vi "VISJS Viewer.vi"(4 "Extra Scripts":string, 5 "FileDependency out":map{path, T1}(c390), 6 "Options":string, 7 "OpenWebBrowser(False)":bool, 8 "error in":errorcluster, 9 "Embedd VISJS Librarya in HTMl File(False)":bool, 10 "HTMLFilePath":path, 11 "LibraryDependency":map{path, T3}(c390)) -> (0 "error out":errorcluster, 3 "HTMLFileContent":string)   [LabVIEW 2020, in "VISJS Viewer.lvlib"] (continued)
this.defaultOptions),this.body.emitter.on(\"_dataChanged\",(function(){e.updateSelection()}))}return kd(g,[{key:\"setOptions\",value:function(g){if(void 0!==g){Xf([\"multiselect\",\"hoverConnectedEdges\",\"selectable\",\"selectConnectedEdges\"],this.options,g)}}},{key:\"selectOnPoint\",value:function(g){var t=!1;if(!0===this.options.selectable){var A=this.getNodeAt(g)||this.getEdgeAt(g);this.unselectAll(),void 0!==A&&(t=this.selectObject(A)),this.body.emitter.emit(\"_requestRedraw\")}return t}},{key:\"selectAdditionalOnPoint\",value:function(g){var t=!1;if(!0===this.options.selectable){var A=this.getNodeAt(g)||this.getEdgeAt(g);void 0!==A&&(t=!0,!0===A.isSelected()?this.deselectObject(A):this.selectObject(A),this.body.emitter.emit(\"_requestRedraw\"))}return t}},{key:\"_initBaseEvent\",value:function(g,t){var A={};return A.pointer={DOM:{x:t.x,y:t.y},canvas:this.canvas.DOMtoCanvas(t)},A.event=g,A}},{key:\"generateClickEvent\",value:function(g,t,A,e){var C=arguments.length>4&&void 0!==arguments[4]&&arguments[4],I=this._initBaseEvent(t,A);if(!0===C)I.nodes=[],I.edges=[];else{var i=this.getSelection();I.nodes=i.nodes,I.edges=i.edges}void 0!==e&&(I.previousSelection=e),\"click\"==g&&(I.items=this.getClickedItems(A)),void 0!==t.controlEdge&&(I.controlEdge=t.controlEdge),this.body.emitter.emit(g,I)}},{key:\"selectObject\",value:function(g){var t=arguments.length>1&&void 0!==arguments[1]?arguments[1]:this.options.selectConnectedEdges;if(void 0!==g){if(g instanceof jN){var A;if(!0===t)(A=this._selectionAccumulator).addEdges.apply(A,ch(g.edges));this._selectionAccumulator.addNodes(g)}else this._selectionAccumulator.addEdges(g);return!0}return!1}},{key:\"deselectObject\",value:function(g){!0===g.isSelected()&&(g.selected=!1,this._removeFromSelection(g))}},{key:\"_getAllNodesOverlappingWith\",value:function(g){for(var t=[],A=this.body.nodes,e=0;e<this.body.nodeIndices.length;e++){var C=this.body.nodeIndices[e];A[C].isOverlappingWith(g)&&t.push(C)}return t}},{key:\"_pointerToPositionObject\",value:function(g){var t=this.canvas.DOMtoCanvas(g);return{left:t.x-1,top:t.y+1,right:t.x+1,bottom:t.y-1}}},{key:\"getNodeAt\",value:function(g){var t=!(arguments.length>1&&void 0!==arguments[1])||arguments[1],A=this._pointerToPositionObject(g),e=this._getAllNodesOverlappingWith(A);return e.length>0?!0===t?this.body.nodes[e[e.length-1]]:e[e.length-1]:void 0}},{key:\"_getEdgesOverlappingWith\",value:function(g,t){for(var A=this.body.edges,e=0;e<this.body.edgeIndices.length;e++){var C=this.body.edgeIndices[e];A[C].isOverlappingWith(g)&&t.push(C)}}},{key:\"_getAllEdgesOverlappingWith\",value:function(g){var t=[];return this._getEdgesOverlappingWith(g,t),t}},{key:\"getEdgeAt\",value:function(g){for(var t=!(arguments.length>1&&void 0!==arguments[1])||arguments[1],A=this.canvas.DOMtoCanvas(g),e=10,C=null,I=this.body.edges,i=0;i<this.body.edgeIndices.length;i++){var o=this.body.edgeIndices[i],n=I[o];if(n.connected){var r=n.from.x,s=n.from.y,a=n.to.x,d=n.to.y,h=n.edgeType.getDistanceToEdge(r,s,a,d,A.x,A.y);h<e&&(C=o,e=h)}}return null!==C?!0===t?this.body.edges[C]:C:void 0}},{key:\"_addToHover\",value:function(g){g instanceof jN?this.hoverObj.nodes[g.id]=g:this.hoverObj.edges[g.id]=g}},{key:\"_removeFromSelection\",value:function(g){var t;g instanceof jN?(this._selectionAccumulator.deleteNodes(g),(t=this._selectionAccumulator).deleteEdges.apply(t,ch(g.edges))):this._selectionAccumulator.deleteEdges(g)}},{key:\"unselectAll\",value:function(){this._selectionAccumulator.clear()}},{key:\"getSelectedNodeCount\",value:function(){return this._selectionAccumulator.sizeNodes}},{key:\"getSelectedEdgeCount\",value:function(){return this._selectionAccumulator.sizeEdges}},{key:\"_hoverConnectedEdges\",value:function(g){for(var t=0;t<g.edges.length;t++){var A=g.edges[t];A.hover=!0,this._addToHover(A)}}},{key:\"emitBlurEvent\",value:function(g,t,A){var e=this._initBaseEvent(g,t);!0===A.hover&&(A.hover=!1,A instanceof jN?(e.node=A.id,this.body.emitter.emit(\"blurNode\",e)):(e.edge=A.id,this.body.emitter.emit(\"blurEdge\",e)))}},{key:\"emitHoverEvent\",value:function(g,t,A){var e=this._initBaseEvent(g,t),C=!1;return!1===A.hover&&(A.hover=!0,this._addToHover(A),C=!0,A instanceof jN?(e.node=A.id,this.body.emitter.emit(\"hoverNode\",e)):(e.edge=A.id,this.body.emitter.emit(\"hoverEdge\",e))),C}},{key:\"hoverObject\",value:function(g,t){var A=this.getNodeAt(t);void 0===A&&(A=this.getEdgeAt(t));var e=!1;for(var C in this.hoverObj.nodes)Object.prototype.hasOwnProperty.call(this.hoverObj.nodes,C)&&(void 0===A||A instanceof jN&&A.id!=C||A instanceof ZR)&&(this.emitBlurEvent(g,t,this.hoverObj.nodes[C]),delete this.hoverObj.nodes[C],e=!0);for(var I in this.hoverObj.edges)Object.prototype.hasOwnProperty.call(this.hoverObj.edges,I)&&(!0===e?(this.hoverObj.edges[I].hover=!1,delete this.hoverObj.edges[I]):(void 0===A||A instanceof ZR&&A.id!=I||A instanceof jN&&!A.hover)&&(this.emitBlurEvent(g,t,this.hoverObj.edges[I]),delete this.hoverObj.edges[I],e=!0));if(void 0!==A){var i=Lh(this.hoverObj.edges).length,o=Lh(this.hoverObj.nodes).length;(e||A instanceof ZR&&0===i&&0===o||A instanceof jN&&0===i&&0===o)&&(e=this.emitHoverEvent(g,t,A)),A instanceof jN&&!0===this.options.hoverConnectedEdges&&this._hoverConnectedEdges(A)}!0===e&&this.body.emitter.emit(\"_requestRedraw\")}},{key:\"commitWithoutEmitting\",value:function(){this._selectionAccumulator.commit()}},{key:\"commitAndEmit\",value:function(g,t){var A=!1,e=this._selectionAccumulator.commit(),C={nodes:e.nodes.previous,edges:e.edges.previous};e.edges.deleted.length>0&&(this.generateClickEvent(\"deselectEdge\",t,g,C),A=!0),e.nodes.deleted.length>0&&(this.generateClickEvent(\"deselectNode\",t,g,C),A=!0),e.nodes.added.length>0&&(this.generateClickEvent(\"selectNode\",t,g),A=!0),e.edges.added.length>0&&(this.generateClickEvent(\"selectEdge\",t,g),A=!0),!0===A&&this.generateClickEvent(\"select\",t,g)}},{key:\"getSelection\",value:function(){return{nodes:this.getSelectedNodeIds(),edges:this.getSelectedEdgeIds()}}},{key:\"getSelectedNodes\",value:function(){return this._selectionAccumulator.getNodes()}},{key:\"getSelectedEdges\",value:function(){return this._selectionAccumulator.getEdges()}},{key:\"getSelectedNodeIds\",value:function(){var g;return Fh(g=this._selectionAccumulator.getNodes()).call(g,(function(g){return g.id}))}},{key:\"getSelectedEdgeIds\",value:function(){var g;return Fh(g=this._selectionAccumulator.getEdges()).call(g,(function(g){return g.id}))}},{key:\"setSelection\",value:function(g){var t=arguments.length>1&&void 0!==arguments[1]?arguments[1]:{};if(!g||!g.nodes&&!g.edges)throw new TypeError(\"Selection must be an object with nodes and/or edges properties\");if((t.unselectAll||void 0===t.unselectAll)&&this.unselectAll(),g.nodes){var A,e=fM(g.nodes);try{for(e.s();!(A=e.n()).done;){var C=A.value,I=this.body.nodes[C];if(!I)throw new RangeError('Node with id \"'+C+'\" not found');this.selectObject(I,t.highlightEdges)}}catch(g){e.e(g)}finally{e.f()}}if(g.edges){var i,o=fM(g.edges);try{for(o.s();!(i=o.n()).done;){var n=i.value,r=this.body.edges[n];if(!r)throw new RangeError('Edge with id \"'+n+'\" not found');this.selectObject(r)}}catch(g){o.e(g)}finally{o.f()}}this.body.emitter.emit(\"_requestRedraw\"),this._selectionAccumulator.commit()}},{key:\"selectNodes\",value:function(g){var t=!(arguments.length>1&&void 0!==arguments[1])||arguments[1];if(!g||void 0===g.length)throw\"Selection must be an array with ids\";this.setSelection({nodes:g},{highlightEdges:t})}},{key:\"selectEdges\",value:function(g){if(!g||void 0===g.length)throw\"Selection must be an array with ids\";this.setSelection({edges:g})}},{key:\"updateSelection\",value:function(){for(var g in this._selectionAccumulator.getNodes())Object.prototype.hasOwnProperty.call(this.body.nodes,g.id)||this._selectionAccumulator.deleteNodes(g);for(var t in this._selectionAccumulator.getEdges())Object.prototype.hasOwnProperty.call(this.body.edges,t.id)||this._selectionAccumulator.deleteEdges(t)}},{key:\"getClickedItems\",value:function(g){for(var t=this.canvas.DOMtoCanvas(g),A=[],e=this.body.nodeIndices,C=this.body.nodes,I=e.length-1;I>=0;I--){var i=C[e[I]].getItemsOnPoint(t);A.push.apply(A,i)}for(var o=this.body.edgeIndices,n=this.body.edges,r=o.length-1;r>=0;r--){var s=n[o[r]].getItemsOnPoint(t);A.push.apply(A,s)}return A}}]),g}();function mM(g){var t=function(){if(\"undefined\"==typeof Reflect||!MT)return!1;if(MT.sham)return!1;if(\"function\"==typeof Proxy)return!0;try{return Boolean.prototype.valueOf.call(MT(Boolean,[],(function(){}))),!0}catch(g){return!1}}();return function(){var A,e=nb(g);if(t){var C=nb(this).constructor;A=MT(e,arguments,C)}else A=e.apply(this,arguments);return Ib(this,A)}}var bM=function(){function g(){cn(this,g)}return kd(g,[{key:\"abstract\",value:function(){throw new Error(\"Can't instantiate abstract class!\")}},{key:\"fake_use\",value:function(){}},{key:\"curveType\",value:function(){return this.abstract()}},{key:\"getPosition\",value:function(g){return this.fake_use(g),this.abstract()}},{key:\"setPosition\",value:function(g,t){var A=arguments.length>2&&void 0!==arguments[2]?arguments[2]:void 0;this.fake_use(g,t,A),this.abstract()}},{key:\"getTreeSize\",value:function(g){return this.fake_use(g),this.abstract()}},{key:\"sort\",value:function(g){this.fake_use(g),this.abstract()}},{key:\"fix\",value:function(g,t){this.fake_use(g,t),this.abstract()}},{key:\"shift\",value:function(g,t){this.fake_use(g,t),this.abstract()}}]),g}(),wM=function(g){Cb(A,g);var t=mM(A);function A(g){var e;return cn(this,A),(e=t.call(this)).layout=g,e}return kd(A,[{key:\"curveType\",value:function(){return\"horizontal\"}},{key:\"getPosition\",value:function(g){return g.x}},{key:\"setPosition\",value:function(g,t){var A=arguments.length>2&&void 0!==arguments[2]?arguments[2]:void 0;void 0!==A&&this.layout.hierarchical.addToOrdering(g,A),g.x=t}},{key:\"getTreeSize\",value:function(g){var t=this.layout.hierarchical.getTreeSize(this.layout.body.nodes,g);return{min:t.min_x,max:t.max_x}}},{key:\"sort\",value:function(g){WO(g).call(g,(function(g,t){return g.x-t.x}))}},{key:\"fix\",value:function(g,t){g.y=this.layout.options.hierarchical.levelSeparation*t,g.options.fixed.y=!0}},{key:\"shift\",value:function(g,t){this.layout.body.nodes[g].x+=t}}]),A}(bM),kM=function(g){Cb(A,g);var t=mM(A);function A(g){var e;return cn(this,A),(e=t.call(this)).layout=g,e}return kd(A,[{key:\"curveType\",value:function(){return\"vertical\"}},{key:\"getPosition\",value:function(g){return g.y}},{key:\"setPosition\",value:function(g,t){var A=arguments.length>2&&void 0!==arguments[2]?arguments[2]:void 0;void 0!==A&&this.layout.hierarchical.addToOrdering(g,A),g.y=t}},{key:\"getTreeSize\",value:function(g){var t=this.layout.hierarchical.getTreeSize(this.layout.body.nodes,g);return{min:t.min_y,max:t.max_y}}},{key:\"sort\",value:function(g){WO(g).call(g,(function(g,t){return g.y-t.y}))}},{key:\"fix\",value:function(g,t){g.x=this.layout.options.hierarchical.levelSeparation*t,g.options.fixed.x=!0}},{key:\"shift\",value:function(g,t){this.layout.body.nodes[g].y+=t}}]),A}(bM),xM=Sr.every;TA({target:\"Array\",proto:!0,forced:!_h(\"every\")},{every:function(g){return xM(this,g,arguments.length>1?arguments[1]:void 0)}});var EM=Me(\"Array\").every,OM=og,TM=EM,DM=Array.prototype,NM=function(g){var t=g.every;return g===DM||OM(DM,g)&&t===DM.every?TM:t},RM=A(NM);function PM(g,t){var A=void 0!==uh&&ln(g)||g[\"@@iterator\"];if(!A){if(Rh(g)||(A=function(g,t){var A;if(!g)return;if(\"string\"==typeof g)return MM(g,t);var e=wh(A=Object.prototype.toString.call(g)).call(A,8,-1);\"Object\"===e&&g.constructor&&(e=g.constructor.name);if(\"Map\"===e||\"Set\"===e)return Uo(g);if(\"Arguments\"===e||/^(?:Ui|I)nt(?:8|16|32)(?:Clamped)?Array$/.test(e))return MM(g,t)}(g))||t&&g&&\"number\"==typeof g.length){A&&(g=A);var e=0,C=function(){};return{s:C,n:function(){return e>=g.length?{done:!0}:{done:!1,value:g[e++]}},e:function(g){throw g},f:C}}throw new TypeError(\"Invalid attempt to iterate non-iterable instance.\\nIn order to be iterable, non-array objects must have a [Symbol.iterator]() method.\")}var I,i=!0,o=!1;return{s:function(){A=A.call(g)},n:function(){var g=A.next();return i=g.done,g},e:function(g){o=!0,I=g},f:function(){try{i||null==A.return||A.return()}finally{if(o)throw I}}}}function MM(g,t){(null==t||t>g.length)&&(t=g.length);for(var A=0,e=new Array(t);A<t;A++)e[A]=g[A];return e}function BM(g,t){var A=new CO;return Cl(g).call(g,(function(g){var t;Cl(t=g.edges).call(t,(function(g){g.connected&&A.add(g)}))})),Cl(A).call(A,(function(g){var A=g.from.id,e=g.to.id;null==t[A]&&(t[A]=0),(null==t[e]||t[A]>=t[e])&&(t[e]=t[A]+1)})),t}function zM(g,t,A,e){var C,I,i=$c(null),o=LE(C=ch(nT(e).call(e))).call(C,(function(g,t){return g+1+t.edges.length}),0),n=A+\"Id\",r=\"to\"===A?1:-1,s=PM(e);try{var a,d=function(){var C=lh(I.value,2),s=C[0],a=C[1];if(!e.has(s)||!g(a))return 0;i[s]=0;for(var d,h,l=[a],c=0,u=function(){var g,C;if(!e.has(s))return 0;var I=i[d.id]+r;if(Cl(g=pc(C=d.edges).call(C,(function(g){return g.connected&&g.to!==g.from&&g[A]!==d&&e.has(g.toId)&&e.has(g.fromId)}))).call(g,(function(g){var e=g[n],C=i[e];(null==C||t(I,C))&&(i[e]=I,l.push(g[A]))})),c>o)return{v:{v:BM(e,i)}};++c};d=l.pop();)if(0!==(h=u())&&h)return h.v};for(s.s();!(I=s.n()).done;)if(0!==(a=d())&&a)return a.v}catch(g){s.e(g)}finally{s.f()}return i}var SM=function(){function g(){cn(this,g),this.childrenReference={},this.parentReference={},this.trees={},this.distributionOrdering={},this.levels={},this.distributionIndex={},this.isTree=!1,this.treeIndex=-1}return kd(g,[{key:\"addRelation\",value:function(g,t){void 0===this.childrenReference[g]&&(this.childrenReference[g]=[]),this.childrenReference[g].push(t),void 0===this.parentReference[t]&&(this.parentReference[t]=[]),this.parentReference[t].push(g)}},{key:\"checkIfTree\",value:function(){for(var g in this.parentReference)if(this.parentReference[g].length>1)return void(this.isTree=!1);this.isTree=!0}},{key:\"numTrees\",value:function(){return this.treeIndex+1}},{key:\"setTreeIndex\",value:function(g,t){void 0!==t&&void 0===this.trees[g.id]&&(this.trees[g.id]=t,this.treeIndex=Math.max(t,this.treeIndex))}},{key:\"ensureLevel\",value:function(g){void 0===this.levels[g]&&(this.levels[g]=0)}},{key:\"getMaxLevel\",value:function(g){var t=this,A={};return function g(e){if(void 0!==A[e])return A[e];var C=t.levels[e];if(t.childrenReference[e]){var I=t.childrenReference[e];if(I.length>0)for(var i=0;i<I.length;i++)C=Math.max(C,g(I[i]))}return A[e]=C,C}(g)}},{key:\"levelDownstream\",value:function(g,t){void 0===this.levels[t.id]&&(void 0===this.levels[g.id]&&(this.levels[g.id]=0),this.levels[t.id]=this.levels[g.id]+1)}},{key:\"setMinLevelToZero\",value:function(g){var t=1e9;for(var A in g)Object.prototype.hasOwnProperty.call(g,A)&&void 0!==this.levels[A]&&(t=Math.min(this.levels[A],t));for(var e in g)Object.prototype.hasOwnProperty.call(g,e)&&void 0!==this.levels[e]&&(this.levels[e]-=t)}},{key:\"getTreeSize\",value:function(g,t){var A=1e9,e=-1e9,C=1e9,I=-1e9;for(var i in this.trees)if(Object.prototype.hasOwnProperty.call(this.trees,i)&&this.trees[i]===t){var o=g[i];A=Math.min(o.x,A),e=Math.max(o.x,e),C=Math.min(o.y,C),I=Math.max(o.y,I)}return{min_x:A,max_x:e,min_y:C,max_y:I}}},{key:\"hasSameParent\",value:function(g,t){var A=this.parentReference[g.id],e=this.parentReference[t.id];if(void 0===A||void 0===e)return!1;for(var C=0;C<A.length;C++)for(var I=0;I<e.length;I++)if(A[C]==e[I])return!0;return!1}},{key:\"inSameSubNetwork\",value:function(g,t){return this.trees[g.id]===this.trees[t.id]}},{key:\"getLevels\",value:function(){return Lh(this.distributionOrdering)}},{key:\"addToOrdering\",value:function(g,t){void 0===this.distributionOrdering[t]&&(this.distributionOrdering[t]=[]);var A=!1,e=this.distributionOrdering[t];for(var C in e)if(e[C]===g){A=!0;break}A||(this.distributionOrdering[t].push(g),this.distributionIndex[g.id]=this.distributionOrdering[t].length-1)}}]),g}(),ZM=function(){function g(t){cn(this,g),this.body=t,this._resetRNG(Math.random()+\":\"+Qh()),this.setPhysics=!1,this.options={},this.optionsBackup={physics:{}},this.defaultOptions={randomSeed:void 0,improvedLayout:!0,clusterThreshold:150,hierarchical:{enabled:!1,levelSeparation:150,nodeSpacing:100,treeSpacing:200,blockShifting:!0,edgeMinimization:!0,parentCentralization:!0,direction:\"UD\",sortMethod:\"hubsize\"}},fe(this.options,this.defaultOptions),this.bindEventListeners()}return kd(g,[{key:\"bindEventListeners\",value:function(){var g=this;this.body.emitter.on(\"_dataChanged\",(function(){g.setupHierarchicalLayout()})),this.body.emitter.on(\"_dataLoaded\",(function(){g.layoutNetwork()})),this.body.emitter.on(\"_resetHierarchicalLayout\",(function(){g.setupHierarchicalLayout()})),this.body.emitter.on(\"_adjustEdgesForHierarchicalLayout\",(function(){if(!0===g.options.hierarchical.enabled){var t=g.direction.curveType();g.body.emitter.emit(\"_forceDisableDynamicCurves\",t,!1)}}))}},{key:\"setOptions\",value:function(g,t){if(void 0!==g){var A=this.options.hierarchical,e=A.enabled;if(Xf([\"randomSeed\",\"improvedLayout\",\"clusterThreshold\"],this.options,g),dv(this.options,g,\"hierarchical\"),void 0!==g.randomSeed&&this._resetRNG(g.randomSeed),!0===A.enabled)return!0===e&&this.body.emitter.emit(\"refresh\",!0),\"RL\"===A.direction||\"DU\"===A.direction?A.levelSeparation>0&&(A.levelSeparation*=-1):A.levelSeparation<0&&(A.levelSeparation*=-1),this.setDirectionStrategy(),this.body.emitter.emit(\"_resetHierarchicalLayout\"),this.adaptAllOptionsForHierarchicalLayout(t);if(!0===e)return this.body.emitter.emit(\"refresh\"),qf(t,this.optionsBackup)}return t}},{key:\"_resetRNG\",value:function(g){this.initialRandomSeed=g,this._rng=Ff(this.initialRandomSeed)}},{key:\"adaptAllOptionsForHierarchicalLayout\",value:function(g){if(!0===this.options.hierarchical.enabled){var t=this.optionsBackup.physics;void 0===g.physics||!0===g.physics?(g.physics={enabled:void 0===t.enabled||t.enabled,solver:\"hierarchicalRepulsion\"},t.enabled=void 0===t.enabled||t.enabled,t.solver=t.solver||\"barnesHut\"):\"object\"===yd(g.physics)?(t.enabled=void 0===g.physics.enabled||g.physics.enabled,t.solver=g.physics.solver||\"barnesHut\",g.physics.solver=\"hierarchicalRepulsion\"):!1!==g.physics&&(t.solver=\"barnesHut\",g.physics={solver:\"hierarchicalRepulsion\"});var A=this.direction.curveType();if(void 0===g.edges)this.optionsBackup.edges={smooth:{enabled:!0,type:\"dynamic\"}},g.edges={smooth:!1};else if(void 0===g.edges.smooth)this.optionsBackup.edges={smooth:{enabled:!0,type:\"dynamic\"}},g.edges.smooth=!1;else if(\"boolean\"==typeof g.edges.smooth)this.optionsBackup.edges={smooth:g.edges.smooth},g.edges.smooth={enabled:g.edges.smooth,type:A};else{var e=g.edges.smooth;void 0!==e.type&&\"dynamic\"!==e.type&&(A=e.type),this.optionsBackup.edges={smooth:{enabled:void 0===e.enabled||e.enabled,type:void 0===e.type?\"dynamic\":e.type,roundness:void 0===e.roundness?.5:e.roundness,forceDirection:void 0!==e.forceDirection&&e.forceDirection}},g.edges.smooth={enabled:void 0===e.enabled||e.enabled,type:A,roundness:void 0===e.roundness?.5:e.roundness,forceDirection:void 0!==e.forceDirection&&e.forceDirection}}this.body.emitter.emit(\"_forceDisableDynamicCurves\",A)}return g}},{key:\"positionInitially\",value:function(g){if(!0!==this.options.hierarchical.enabled){this._resetRNG(this.initialRandomSeed);for(var t=g.length+50,A=0;A<g.length;A++){var e=g[A],C=2*Math.PI*this._rng();void 0===e.x&&(e.x=t*Math.cos(C)),void 0===e.y&&(e.y=t*Math.sin(C))}}}},{key:\"layoutNetwork\",value:function(){if(!0!==this.options.hierarchical.enabled&&!0===this.options.improvedLayout){for(var g=this.body.nodeIndices,t=0,A=0;A<g.length;A++){!0===this.body.nodes[g[A]].predefinedPosition&&(t+=1)}if(t<.5*g.length){var e=0,C=this.options.clusterThreshold,I={clusterNodeProperties:{shape:\"ellipse\",label:\"\",group:\"\",font:{multi:!1}},clusterEdgeProperties:{label:\"\",font:{multi:!1},smooth:{enabled:!1}}};if(g.length>C){for(var i=g.length;
